vi "Unreserve Session.vi"(6 "contextId":T4, 8 "error in":errorcluster, 9 "timeout (ms)":i32=-1, 10 "Session Info":T1, 11 "gRPC ID":T4) -> (0 "error out":errorcluster, 3 "gRPC ID out":T4)   [LabVIEW 2020, in "Keysight 34401A DMM Measurement.lvlib"]
uses:
  Keysight 34401A DMM Measurement.lvlib
  <vilib>/gRPC/LabVIEW gRPC Library/Shared/grpcId.ctl
  <vilib>/MeasurementLink/MeasurementLink Session Management Client/RPC Messages/ni_measurementlink_sessionmanagement_v1_SessionInformation.ctl
  <vilib>/MeasurementLink/MeasurementLink Session Management Client/RPC Messages/nidevice_grpc_Session.ctl
  <vilib>/MeasurementLink/MeasurementLink Session Management Client/RPC Messages/ni_measurementlink_sessionmanagement_v1_ChannelMapping.ctl
  <vilib>/MeasurementLink/MeasurementLink Session Management Client/RPC Messages/ni_measurementlink_sessionmanagement_v1_UnreserveSessionsRequest.ctl
  <vilib>/MeasurementLink/MeasurementLink Session Management Client/MeasurementLink Session Management Client.lvlib
  <vilib>/gRPC/LabVIEW gRPC Library/grpc-lvsupport-release.lvlib
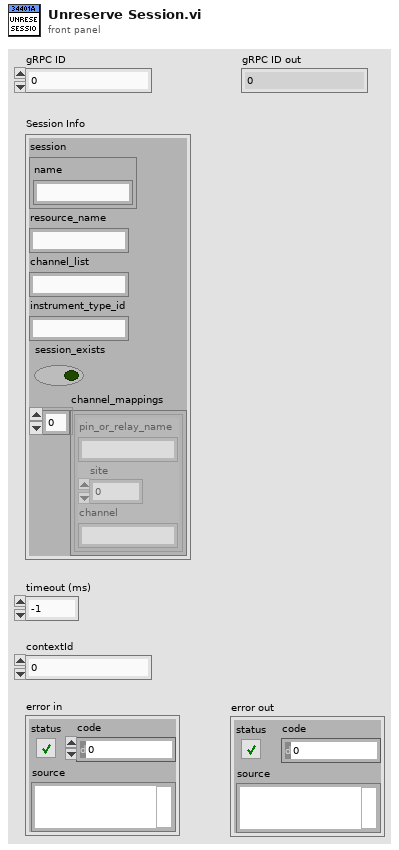
[diagram p1: front panel]
types:
  T1 = typedef "MeasurementLink Session Management Client.lvlib/ni_measurementlink_sessionmanagement_v1_SessionInformation.ctl" = cluster{"session":T2, "resource_name":string, "channel_list":string, "instrument_type_id":string, "session_exists":bool, "channel_mappings":T3[]}
  T2 = typedef "MeasurementLink Session Management Client.lvlib/nidevice_grpc_Session.ctl" = cluster{"name":string}
  T3 = typedef "MeasurementLink Session Management Client.lvlib/ni_measurementlink_sessionmanagement_v1_ChannelMapping.ctl" = cluster{"pin_or_relay_name":string, "site":i32, "channel":string}
  T4 = typedef "grpc-lvsupport-release.lvlib/grpcId.ctl" = u64
  T5 = typedef "MeasurementLink Session Management Client.lvlib/ni_measurementlink_sessionmanagement_v1_UnreserveSessionsRequest.ctl" = cluster{"sessions":T1[]}
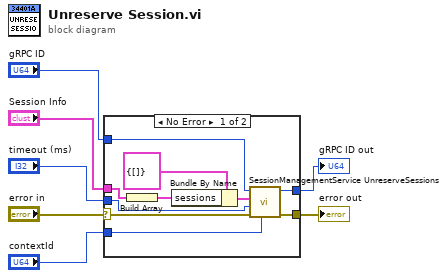
[diagram p0: block diagram]
diagram:
  n1 = case shown="No Error" "error in" {
    selector: "error in" -> [w10 w18]
    tunnel: [w9 w18] -> w6
    tunnel: "gRPC ID" -> [w13 w19]
    tunnel: [w8 w19] -> w4
    tunnel: "timeout (ms)" -> [w11 _]
    tunnel: "contextId" -> [w12 _]
    tunnel: "Session Info" -> [w16 _]
    frame No Error {
      n2 = Build Array(w16) -> (w15:T1[])
      n3 = Bundle By Name(cluster=T5 {"sessions"=[]} ("Request Data"), "sessions"=w15) -> (w14:T5)
      n4 = call <vilib>:"SessionManagementService UnreserveSessions.vi"("contextId"=w12, "error in"=w10, "timeout (ms)"=w11, "Request Data"=w14, "gRPC ID"=w13) -> ("error out"=w9:errorcluster, "gRPC ID out"=w8:T4)  [unwired: 4 in, 1 out]
    }
    frame Error {
    }
  }
  "error out" <- w6
  "gRPC ID out" <- w4
